vi "sedSpectrometer_monitorCommand_enterControl.vi"(8 "error in (no error)":errorcluster, 11 "command_enterControl_Ctl":T1) -> (0 "error out":errorcluster, 2 "function return":i32, 3 "command_enterControl_Ctl out":T1)   [LabVIEW 2016, in "SALLV_sedSpectrometer.lvlib"]
doc: "int sedSpectrometer_shm_monitorCommand_enterControlLV(sedSpectrometer_command_enterControlLV *command_enterControl_Ctl );"
uses:
  SALLV_sedSpectrometer.lvlib
  DataTypes/command_enterControl.ctl
  SALLV_sedSpectrometer.so
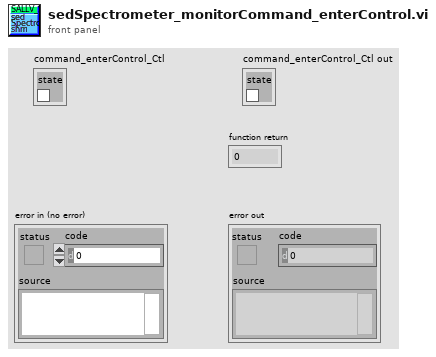
[diagram p1: front panel]
types:
  T1 = typedef "SALLV_sedSpectrometer.lvlib/command_enterControl.ctl" = cluster{"state":bool}
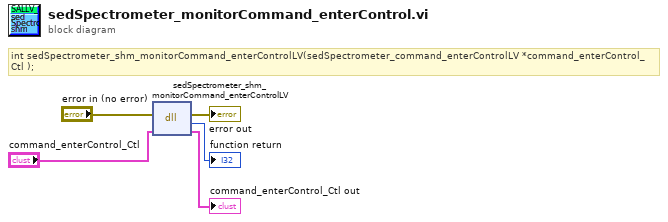
[diagram p0: block diagram]
diagram:
  # "int sedSpectrometer_shm_monitorCommand_enterControlLV(sedSpectrometer_command_enterControlLV *command_enterControl_Ctl );"
  n1 = dll-call lib="home/harini/TCS/ts_sallv_sedSpectrometer/SALLV_sedSpectrometer.*" fn="sedSpectrometer_shm_monitorCommand_enterControlLV"(error in="error in (no error)", "command_enterControl_Ctl"="command_enterControl_Ctl") -> (error out=→"error out":errorcluster, →"function return":i32, "command_enterControl_Ctl"=→"command_enterControl_Ctl out":T1)  [unwired: 2 in, 1 out]
